vi "RichToFlatni_measurementlink_discovery_v1_RegisterServiceResponse.vi"(5 "OutputClusterType":T1, 11 "InputCluster":T2) -> (3 "OutputCluster":T1)   [LabVIEW 2020, in "ni.measurementlink.discovery.v1.api.lvlib"]
uses:
  ni.measurementlink.discovery.v1.api.lvlib
  ni_measurementlink_discovery_v1_RegisterServiceResponse.ctl
  ni_measurementlink_discovery_v1_RegisterServiceResponse_Flat.ctl
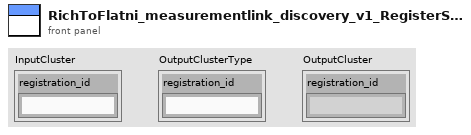
[diagram p1: front panel]
types:
  T1 = typedef "ni.measurementlink.discovery.v1.api.lvlib/ni_measurementlink_discovery_v1_RegisterServiceResponse_Flat.ctl" = cluster{"registration_id":string}
  T2 = typedef "ni.measurementlink.discovery.v1.api.lvlib/ni_measurementlink_discovery_v1_RegisterServiceResponse.ctl" = cluster{"registration_id":string}
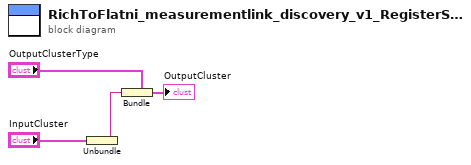
[diagram p0: block diagram]
diagram:
  n1 = Unbundle "Unbundle"("InputCluster") -> ("registration_id"=w1:string)
  n2 = Bundle "Bundle"(cluster="OutputClusterType", "registration_id"=w1) -> (→"OutputCluster":T1)
